vi "从表中获取待查设备.vi"(11 "引用-设备累积管理 i":refnum<vi>) -> (3 "选中的查询设备":string[](array[string]))   [LabVIEW 2017]
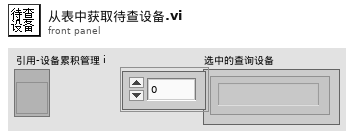
[diagram p1: front panel]
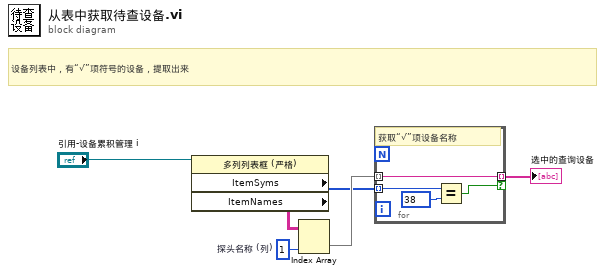
[diagram p0: block diagram]
diagram:
  w5 = 1  # 探头名称 (列)
  # "设备列表中，有“√”项符号的设备，提取出来"
  n1 = property on="属性节点" class="多列列表框 (严格)"(reference="引用-设备累积管理 i") -> ("ItemSyms"=w3:i32[], "ItemNames"=w4:string[][])  [unwired: 1 in, 2 out]
  n2 = Index Array(array=w4, index (col)=w5) -> (element=w6:string[])  [unwired: 1 in]
  n3 = for {
    tunnel: w3 -> [w10] mode=indexing
    tunnel: w6 -> [w8] mode=indexing
    tunnel: [w8] -> w1 mode=indexing if=w7
    # "获取“√”项设备名称"
    n4 = Equal?(x=w10, y=38) -> (x = y?=w7:bool)
  }
  "选中的查询设备" <- w1
